vi "VI Tag(冲突时的文件备份2013-03-27 14-09-45).vi"(7 "Mode":enum16{"Set", "Get", "Get Tag Names"}(ring), 8 "错误输入（无错误）":errorcluster, 9 "Value In":variant, 10 "Tag Name":string, 11 "VI Path":path) -> (0 "错误输出":errorcluster, 1 "Old Value":variant, 3 "Tag Names":string[](array[string]))   [LabVIEW 2012, in "Application.lvlib"]
uses:
  Application.lvlib
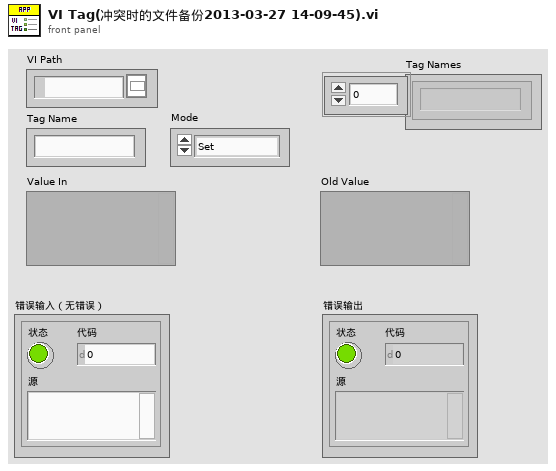
[diagram p1: front panel]
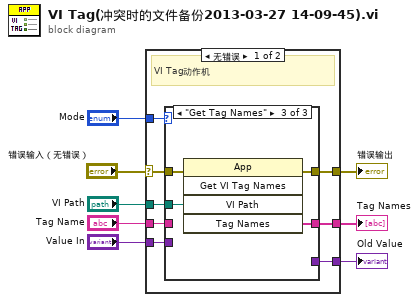
[diagram p0: block diagram]
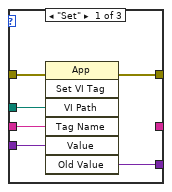
[diagram p2: hidden frame]
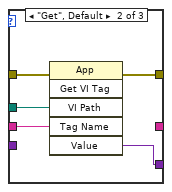
[diagram p3: hidden frame]
diagram:
  n1 = case shown="无错误" "错误输入（无错误）" {
    selector: "错误输入（无错误）" -> [w13 w32]
    tunnel: "Mode" -> [w16 _]
    tunnel: "Tag Name" -> [w15 _]
    tunnel: [w14 _] -> w5
    tunnel: [w12 w32] -> w4
    tunnel: "Value In" -> [w11 _]
    tunnel: "VI Path" -> [w10 _]
    tunnel: [w9 _] -> w1
    frame No Error {
      # "VI Tag动作机"
      n2 = case shown="\"Get Tag Names\"" w16 {
        tunnel: w15 -> [w21 w27 _]
        tunnel: [w17 w26 _] -> w14
        tunnel: w13 -> [w19 w25 w29]
        tunnel: [w18 w24 w30] -> w12
        tunnel: w11 -> [w22 _ _]
        tunnel: w10 -> [w20 w23 w28]
        tunnel: [_ _ w31] -> w9
        frame "Set" {
          # "FGHFD"
          n3 = invoke class="App" method="Set VI Tag"(error in=w19, "VI Path"=w20, "Tag Name"=w21, "Value"=w22) -> (error out=w18:errorcluster, "Old Value"=w17:variant)  [unwired: 3 in, 5 out]
        }
        frame "Get", Default {
          n4 = invoke class="App" method="Get VI Tag"(error in=w25, "VI Path"=w23, "Tag Name"=w27) -> (error out=w24:errorcluster, "Value"=w26:variant)  [unwired: 3 in, 4 out]
        }
        frame "Get Tag Names" {
          n5 = invoke class="App" method="Get VI Tag Names"(error in=w29, "VI Path"=w28) -> (error out=w30:errorcluster, "Tag Names"=w31:string[])  [unwired: 3 in, 3 out]
        }
      }
    }
    frame Error {
    }
  }
  "Tag Names" <- w1
  "错误输出" <- w4
  "Old Value" <- w5
